vi "Init Module.vi"(8 "error in":errorcluster, 11 "Singleton Module Admin in":refnum<class "Delacor_lib_QMH_Module Admin.lvclass">) -> (0 "error out":errorcluster, 1 "Launcher Broadcast Events":T1, 2 "Launcher Request Events":T2, 3 "Singleton Module Admin out":refnum<class "Delacor_lib_QMH_Module Admin.lvclass">)   [LabVIEW 2026, in "Launcher.lvlib"]
doc: "Initialize the module by creating Broadcast Events, Request Events, and synchronization rendezvous.\n_____\nBased on DQMH Dev Tools: Project Template 7.1.2.1547."
uses:
  Launcher.lvlib
  <vilib>/Delacor/Delacor QMH/Libraries/Module Admin_class/Delacor_lib_QMH_Module Admin.lvclass
  Request Events--cluster.ctl
  Stop Argument--cluster.ctl
  Show Panel Argument--cluster.ctl
  Hide Panel Argument--cluster.ctl
  Get Module Execution Status Argument--cluster.ctl
  Show Diagram Argument--cluster.ctl
  Set Captures Folder Argument--cluster.ctl
  Broadcast Events--cluster.ctl
  Did Init Argument--cluster.ctl
  Status Updated Argument--cluster.ctl
  Error Reported Argument--cluster.ctl
  Start Capture Detection Loop Argument--cluster.ctl
  Set Capture Detection Loop Timeout Argument--cluster.ctl
  Trigger Capture Detection Loop Argument--cluster.ctl
  Trigger Capture Detection Loop (Reply Payload)--cluster.ctl
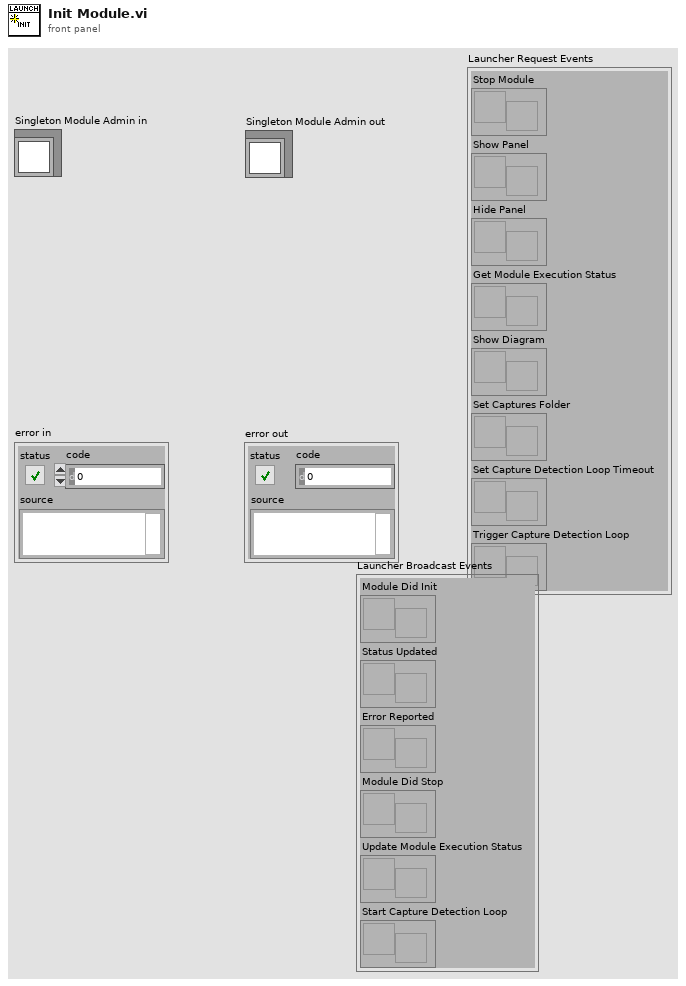
[diagram p1: front panel]
types:
  T1 = typedef "Launcher.lvlib/Broadcast Events--cluster.ctl" = cluster{"Module Did Init":refnum<user-event>, "Status Updated":refnum<user-event>, "Error Reported":refnum<user-event>, "Module Did Stop":refnum<user-event>, "Update Module Execution Status":refnum<user-event>, "Start Capture Detection Loop":refnum<user-event>}
  T2 = typedef "Launcher.lvlib/Request Events--cluster.ctl" = cluster{"Stop Module":refnum<user-event>, "Show Panel":refnum<user-event>, "Hide Panel":refnum<user-event>, "Get Module Execution Status":refnum<user-event>, "Show Diagram":refnum<user-event>, "Set Captures Folder":refnum<user-event>, "Set Capture Detection Loop Timeout":refnum<user-event>, "Trigger Capture Detection Loop":refnum<user-event>}
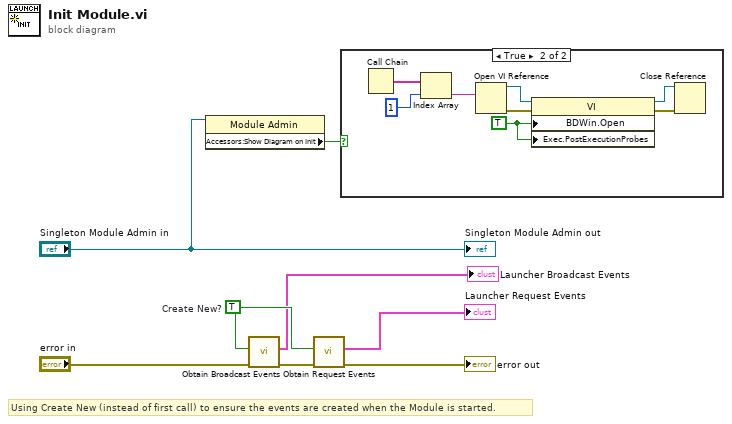
[diagram p0: block diagram]
diagram:
  w5 = TRUE  # Create New?
  # "Using Create New (instead of first call) to ensure the events are created when the Module is started."
  n1 = property class="Module Admin"(reference="Singleton Module Admin in") -> ("Accessors:Show Diagram on Init"=w3:bool)  [unwired: 1 in, 2 out]
  n2 = call "Obtain Broadcast Events.vi"("error in"="error in", "Create New? (F)"=w5) -> ("error out"=w8:errorcluster, "Launcher Broadcast Events"=→"Launcher Broadcast Events":T1)  [unwired: 8 in]
  n3 = call "Obtain Request Events.vi"("error in"=w8, "Create New? (F)"=w5) -> ("error out"=→"error out":errorcluster, "Launcher Request Events"=→"Launcher Request Events":T2)  [unwired: 8 in]
  n4 = case shown="True" w3 {
    frame False {
    }
    frame True {
      w12 = TRUE ("Block Diagram Window:Open")
      n5 = Call Chain() -> (call chain=w16:string[])
      n6 = Index Array(array=w16, index=1) -> (element=w9:string)
      n7 = Open VI Reference(vi path=w9) -> (vi reference=w13:refnum<vi>, error out=w14:errorcluster)  [unwired: 5 in]
      n8 = property class="VI"(reference=w13, error in=w14, "BDWin.Open"=w12, "Exec.PostExecutionProbes"=w12) -> (reference out=w10:refnum<vi>, error out=w11:errorcluster)
      n9 = Close Reference(reference=w10, error in (no error)=w11) -> ()  [unwired: 1 out]
    }
  }
  "Singleton Module Admin out" <- "Singleton Module Admin in"
